vi "BoxcarFilter.vi"(10 "ValuesToAverage":u32=1, 11 "Value":dbl) -> (3 "Output":dbl)   [LabVIEW 2017]
doc: "Averages the last N values and outputs that"
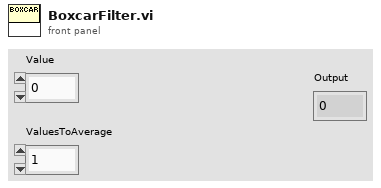
[diagram p1: front panel]
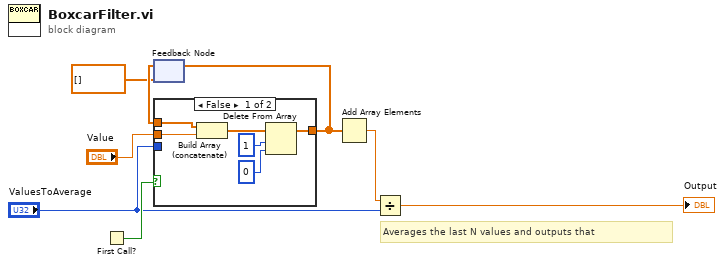
[diagram p0: block diagram]
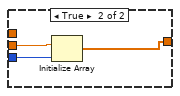
[diagram p2: hidden frame]
diagram:
  # "Averages the last N values and outputs that"
  n1 = First Call?() -> (First Call?: T/F=w8:bool)
  n2 = feedback #1(dbl[] []) -> (w6:dbl[])
  n3 = case shown="False" w8 {
    tunnel: "Value" -> [w13 w17]
    tunnel: "ValuesToAverage" -> [_ w16]
    tunnel: w6 -> [w14 _]
    tunnel: [w11 w15] -> w3
    frame False {
      n4 = Build Array (concatenate)(w14, w13) -> (w12:dbl[])
      n5 = Delete From Array(array=w12, length=1, index=0) -> (array with subset deleted=w11:dbl[])  [unwired: 1 out]
    }
    frame True {
      n6 = Initialize Array(w17, w16) -> (w15:dbl[])
    }
  }
  n7 = feedback-in #1(w3) -> ()
  n8 = Add Array Elements(numeric array=w3) -> (sum=w5:dbl)
  n9 = Divide(x=w5, y="ValuesToAverage") -> (x/y=→"Output":dbl)
